vi "Measurement Core.vi"(8 "error in (no error)":errorcluster, 11 "Servo MSMT in":refnum<class "Servo MSMT.lvclass">) -> (0 "error out":errorcluster, 3 "Servo MSMT out":refnum<class "Servo MSMT.lvclass">)   [LabVIEW 2018, in "Servo MSMT.lvlib" / "Servo MSMT.lvclass"]
uses:
  Servo MSMT.lvclass
  <vilib>/Utility/error.llb/Error Cluster From Error Code.vi
  <vilib>/ErrorRing/Error Ring.xnode
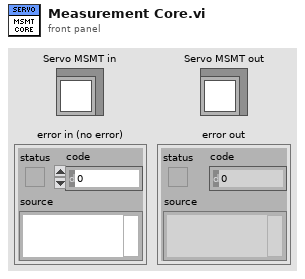
[diagram p1: front panel]
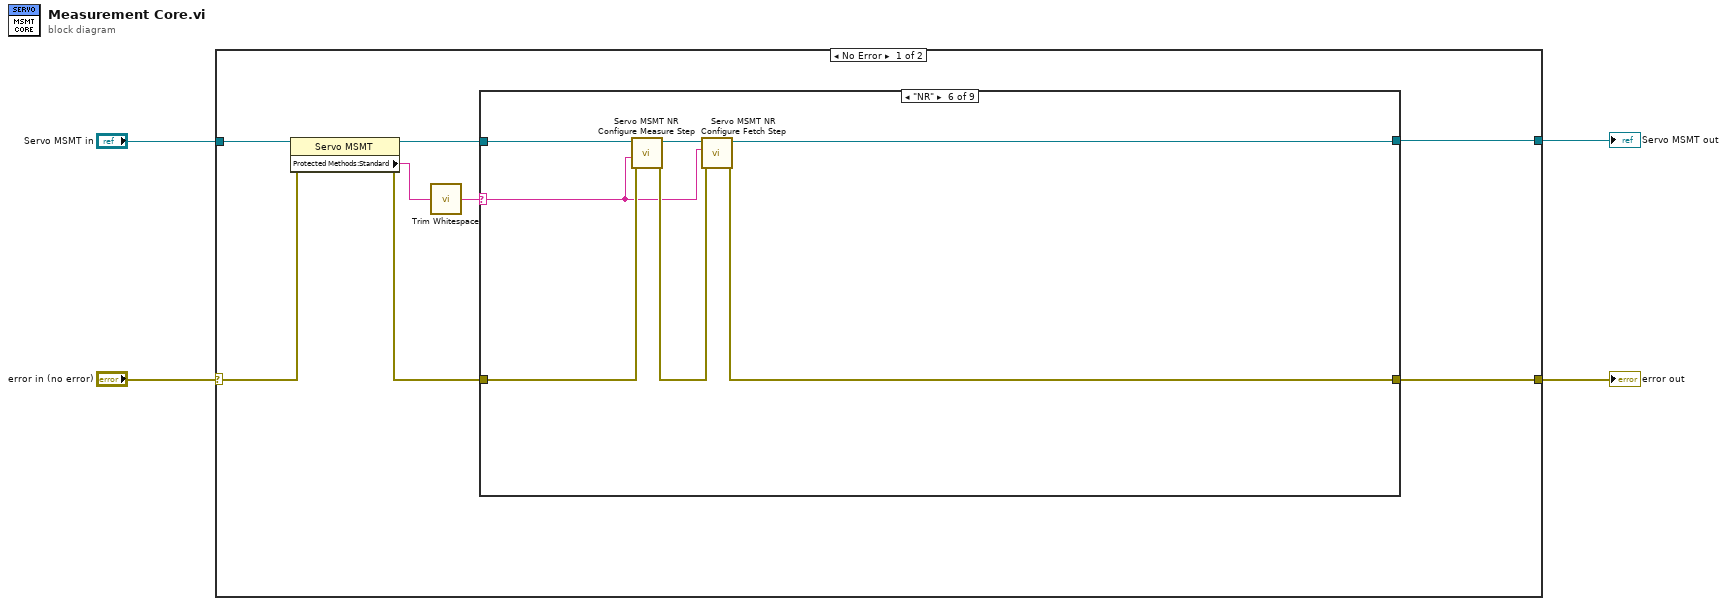
[diagram p0: block diagram]
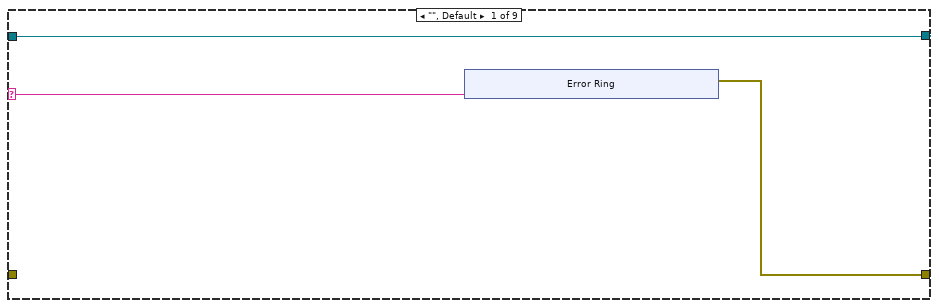
[diagram p2: hidden frame]
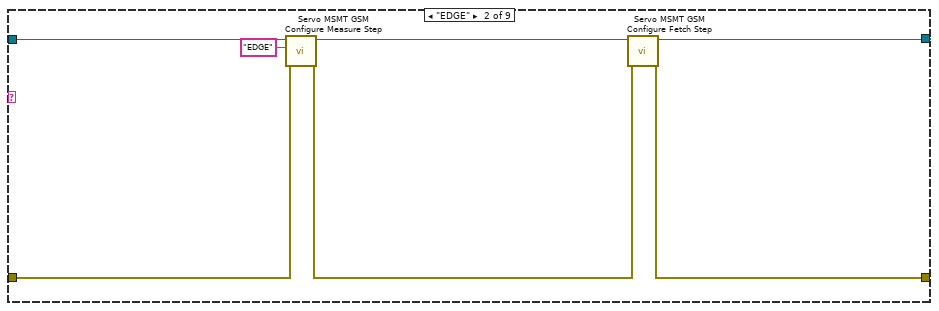
[diagram p3: hidden frame]
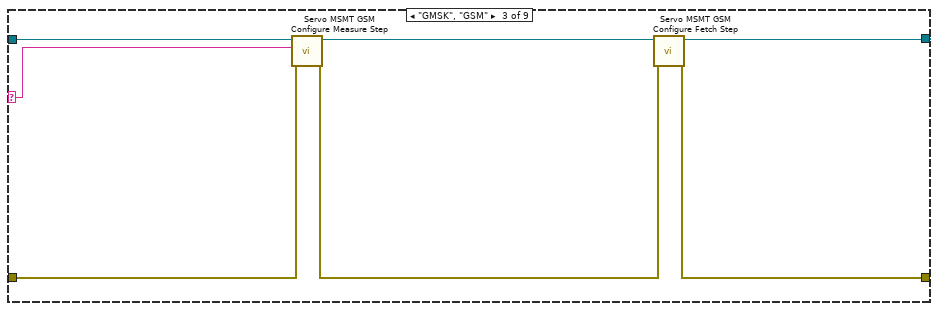
[diagram p4: hidden frame]
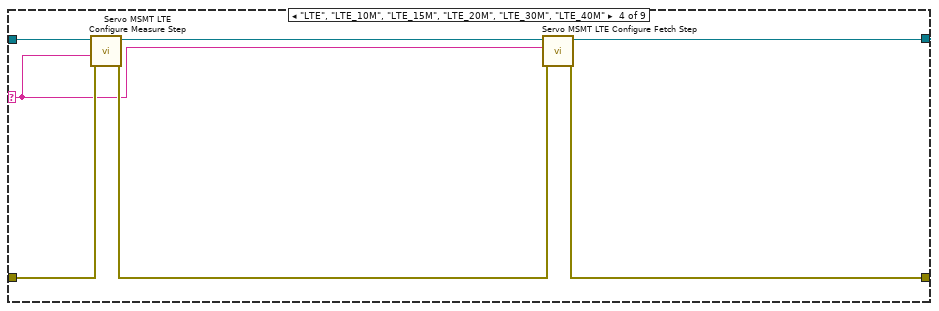
[diagram p5: hidden frame]
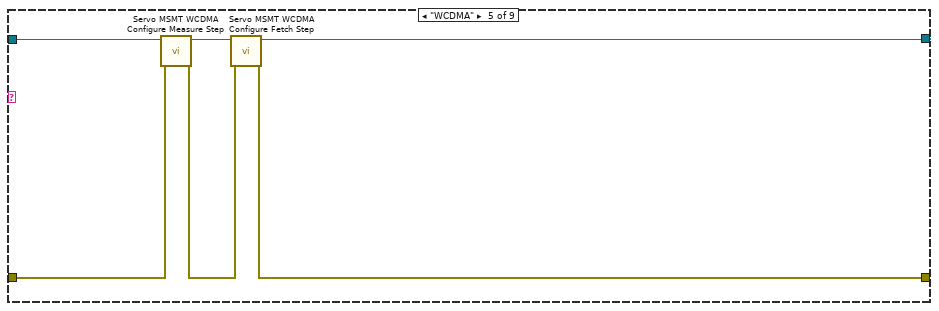
[diagram p6: hidden frame]
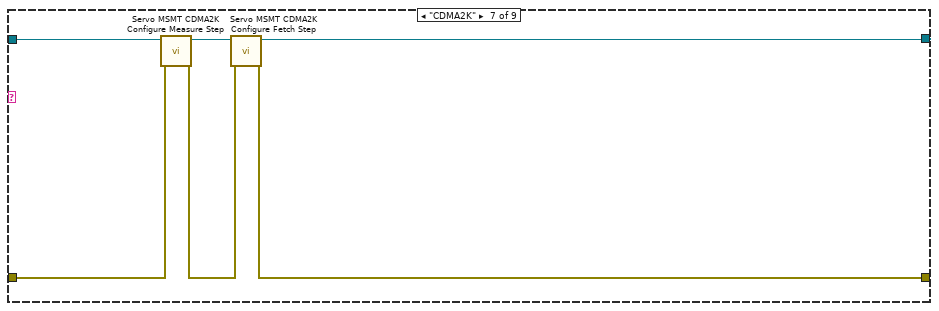
[diagram p7: hidden frame]
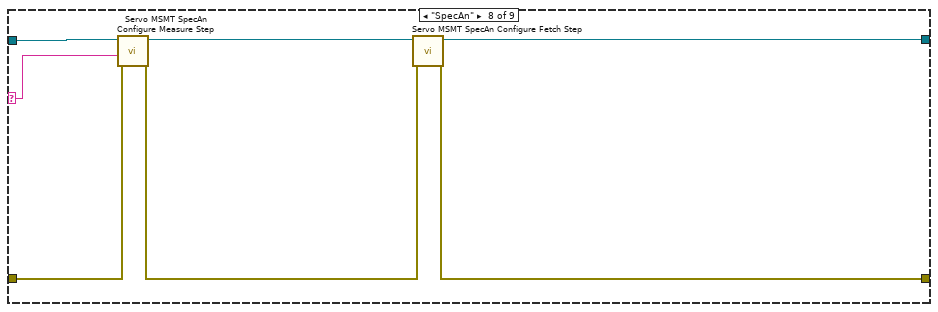
[diagram p8: hidden frame]
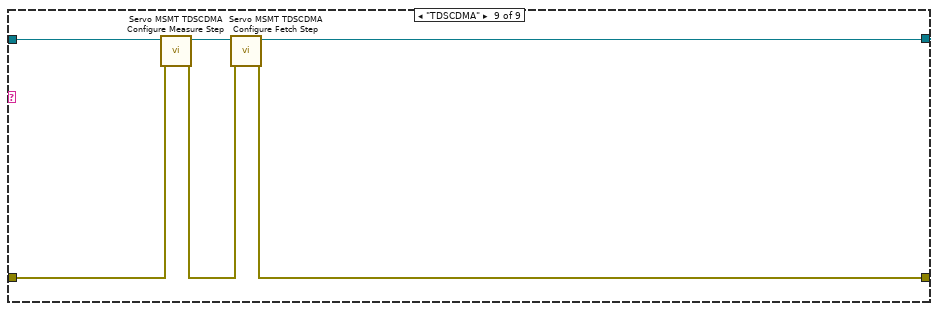
[diagram p9: hidden frame]
diagram:
  n1 = case shown="No Error" "error in (no error)" {
    selector: "error in (no error)" -> [w12 w77]
    tunnel: [w8 w77] -> w3
    tunnel: [w7 w76] -> w1
    tunnel: "Servo MSMT in" -> [w11 w76]
    frame No Error {
      n2 = property class="Servo MSMT"(reference=w11, error in=w12) -> (reference out=w10:refnum<class "Servo MSMT.lvclass">, error out=w9:errorcluster, "Protected Methods:Standard"=w6:string)
      n3 = call <vilib>:"Trim Whitespace.vi"("string"=w6) -> ("trimmed string"=w5:string)  [unwired: 1 in]
      n4 = case shown="\"NR\"" w5 {
        selector: w5 -> [w14 _ w30 w37 _ w50 _ w66 _]
        tunnel: w9 -> [_ w26 w33 w42 w47 w54 w60 w68 w73]
        tunnel: [w15 w27 w34 w38 w44 w51 w57 w63 w70] -> w7
        tunnel: w10 -> [w15 w29 w36 w43 w49 w56 w62 w69 w75]
        tunnel: [w13 w23 w31 w40 w46 w52 w59 w65 w72] -> w8
        frame "", Default {
          n5 = xnode "Error Ring"("parameter 0"=w14) -> ("error out"=w13:errorcluster)
        }
        frame "EDGE" {
          n6 = call "Servo MSMT GSM Configure Measure Step.vi"("error in (no error)"=w26, "Standard"="EDGE", "Servo MSMT in"=w29) -> ("error out"=w24:errorcluster, "Servo MSMT out"=w28:refnum<class "Servo MSMT.lvclass">)  [unwired: 7 in]
          n7 = call "Servo MSMT GSM Configure Fetch Step.vi"("error in (no error)"=w24, "Servo MSMT in"=w28) -> ("error out"=w23:errorcluster, "Servo MSMT out"=w27:refnum<class "Servo MSMT.lvclass">)  [unwired: 8 in]
        }
        frame "GMSK", "GSM" {
          n8 = call "Servo MSMT GSM Configure Measure Step.vi"("error in (no error)"=w33, "Standard"=w30, "Servo MSMT in"=w36) -> ("error out"=w32:errorcluster, "Servo MSMT out"=w35:refnum<class "Servo MSMT.lvclass">)  [unwired: 7 in]
          n9 = call "Servo MSMT GSM Configure Fetch Step.vi"("error in (no error)"=w32, "Servo MSMT in"=w35) -> ("error out"=w31:errorcluster, "Servo MSMT out"=w34:refnum<class "Servo MSMT.lvclass">)  [unwired: 8 in]
        }
        frame "LTE", "LTE_10M", "LTE_15M", "LTE_20M", "LTE_30M", "LTE_40M" {
          n10 = call "Servo MSMT LTE Configure Measure Step.vi"("error in (no error)"=w42, "Standard"=w37, "Servo MSMT in"=w43) -> ("error out"=w41:errorcluster, "Servo MSMT out"=w39:refnum<class "Servo MSMT.lvclass">)  [unwired: 7 in]
          n11 = call "Servo MSMT LTE Configure Fetch Step.vi"("error in (no error)"=w41, "LTE Standard In"=w37, "Servo MSMT in"=w39) -> ("error out"=w40:errorcluster, "Servo MSMT out"=w38:refnum<class "Servo MSMT.lvclass">)  [unwired: 7 in]
        }
        frame "WCDMA" {
          n12 = call "Servo MSMT WCDMA Configure Measure Step.vi"("error in (no error)"=w47, "Servo MSMT in"=w49) -> ("error out"=w48:errorcluster, "Servo MSMT out"=w45:refnum<class "Servo MSMT.lvclass">)  [unwired: 8 in]
          n13 = call "Servo MSMT WCDMA Configure Fetch Step.vi"("error in (no error)"=w48, "Servo MSMT in"=w45) -> ("error out"=w46:errorcluster, "Servo MSMT out"=w44:refnum<class "Servo MSMT.lvclass">)  [unwired: 8 in]
        }
        frame "NR" {
          n14 = call "Servo MSMT NR Configure Measure Step.vi"("error in (no error)"=w54, "Standard"=w50, "Servo MSMT in"=w56) -> ("error out"=w55:errorcluster, "Servo MSMT out"=w53:refnum<class "Servo MSMT.lvclass">)  [unwired: 7 in]
          n15 = call "Servo MSMT NR Configure Fetch Step.vi"("error in (no error)"=w55, "Standard In"=w50, "Servo MSMT in"=w53) -> ("error out"=w52:errorcluster, "Servo MSMT out"=w51:refnum<class "Servo MSMT.lvclass">)  [unwired: 7 in]
        }
        frame "CDMA2K" {
          n16 = call "Servo MSMT CDMA2K Configure Measure Step.vi"("error in (no error)"=w60, "Servo MSMT in"=w62) -> ("error out"=w61:errorcluster, "Servo MSMT out"=w58:refnum<class "Servo MSMT.lvclass">)  [unwired: 8 in]
          n17 = call "Servo MSMT CDMA2K Configure Fetch Step.vi"("error in (no error)"=w61, "Servo MSMT in"=w58) -> ("error out"=w59:errorcluster, "Servo MSMT out"=w57:refnum<class "Servo MSMT.lvclass">)  [unwired: 8 in]
        }
        frame "SpecAn" {
          n18 = call "Servo MSMT SpecAn Configure Measure Step.vi"("error in (no error)"=w68, "Standard"=w66, "Servo MSMT in"=w69) -> ("error out"=w67:errorcluster, "Servo MSMT out"=w64:refnum<class "Servo MSMT.lvclass">)  [unwired: 7 in]
          n19 = call "Servo MSMT SpecAn Configure Fetch Step.vi"("error in (no error)"=w67, "Servo MSMT in"=w64) -> ("error out"=w65:errorcluster, "Servo MSMT out"=w63:refnum<class "Servo MSMT.lvclass">)  [unwired: 8 in]
        }
        frame "TDSCDMA" {
          n20 = call "Servo MSMT TDSCDMA Configure Measure Step.vi"("error in (no error)"=w73, "Servo MSMT in"=w75) -> ("error out"=w74:errorcluster, "Servo MSMT out"=w71:refnum<class "Servo MSMT.lvclass">)  [unwired: 8 in]
          n21 = call "Servo MSMT TDSCDMA Configure Fetch Step.vi"("error in (no error)"=w74, "Servo MSMT in"=w71) -> ("error out"=w72:errorcluster, "Servo MSMT out"=w70:refnum<class "Servo MSMT.lvclass">)  [unwired: 8 in]
        }
      }
    }
    frame Error {
    }
  }
  "error out" <- w3
  "Servo MSMT out" <- w1
